vi "ReflectiveFunc.FitFunc.vi"(3 "output control":T1, 4 "data":variant, 5 "X":dbl[](array[numeric]), 6 "Coefficients":dbl[](array[numeric])) -> (0 "error out":errorcluster, 1 "f'(X,a)":dbl[][](array[numeric]), 2 "f(X,a)":dbl[](array[numeric]))   [LabVIEW 2020, in "XYcenter.lvlib"]
uses:
  XYcenter.lvlib
  <vilib>/gmath/NumericalOptimization/LM_output select.ctl
  <vilib>/gmath/NI_Gmath.lvlib
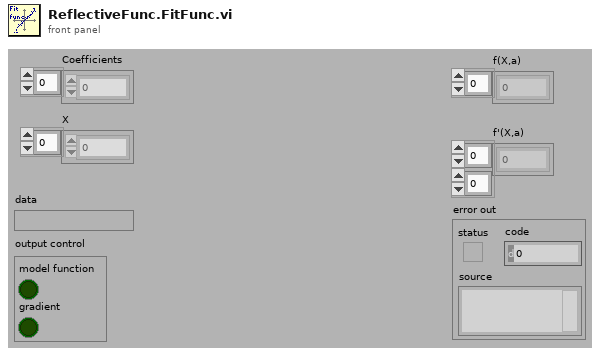
[diagram p1: front panel]
types:
  T1 = typedef "NI_Gmath.lvlib/LM_output select.ctl" = cluster{"model function":bool, "gradient":bool}
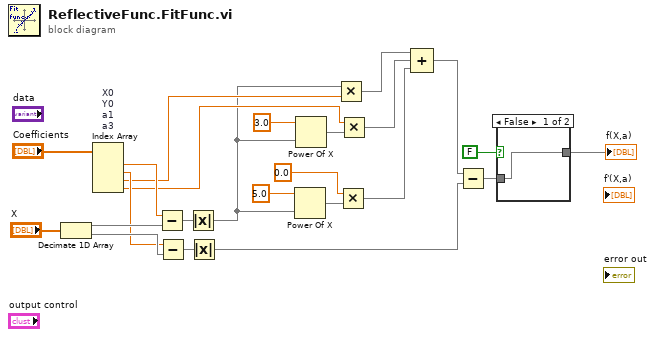
[diagram p0: block diagram]
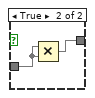
[diagram p2: hidden frame]
diagram:
  n1 = Decimate 1D Array("X") -> (w19:dbl[], w20:dbl[])
  n2 = Index Array "X0\nY0\na1\na3"(array="Coefficients") -> (element #1=w17:dbl, element #2=w18:dbl, element #3=w8:dbl, element #4=w7:dbl)  [unwired: 4 in]
  n3 = Subtract(x=w17, y=w19) -> (x-y=w22:dbl[])
  n4 = Subtract(x=w18, y=w20) -> (x-y=w21:dbl[])
  n5 = Absolute Value(x=w22) -> (abs(x)=w4:dbl[])
  n6 = Absolute Value(x=w21) -> (abs(x)=w12:dbl[])
  n7 = Power Of X(1:w4, 2:5.0) -> (0:w5:dbl[])
  n8 = Power Of X(1:w4, 2:3.0) -> (0:w15:dbl[])
  n9 = Multiply(x=w4, y=w8) -> (x*y=w14:dbl[])
  n10 = Multiply(x=0.0, y=w5) -> (x*y=w3:dbl[])
  n11 = Multiply(x=w7, y=w15) -> (x*y=w9:dbl[])
  n12 = Compound Arithmetic op=ADD(w14, w9, w3) -> (w13:dbl[])
  n13 = Subtract(x=w13, y=w12) -> (x-y=w11:dbl[])
  n14 = case shown="False" FALSE {
    tunnel: w11 -> [w25 w27]
    tunnel: [w25 w26] -> w10
    frame False {
    }
    frame True {
      n15 = Multiply(x=w27, y=w27) -> (x*y=w26:dbl[])
    }
  }
  "f(X,a)" <- w10
